vi "LL_GET Bucket.vi"(4 "Region":T1, 7 "GET Bucket Request Parameters":T9 {"max-keys" max=1000}, 8 "error in (no error)":errorcluster, 9 "Bucket":string, 11 "Headers":T8[](array[typedef])) -> (0 "error out":errorcluster, 1 "Call Result":T2, 3 "ListBucketResult":T3)   [LabVIEW 2015, in "LV Interface for Amazon S3.lvlib"]
doc: "This core implementation of the GET operation returns some or all (up to 1000) of the objects in a bucket. You can use the request parameters as selection criteria to return a subset of the objects in a bucket. You have direct access to HTTP headers, so you can use this VI to implement special requests or API calls not present in this toolkit."
uses:
  LV Interface for Amazon S3.lvlib
  Typedefs/AMZ_S3_API_GET Bucket Request Parameters.ctl
  Typedefs/AMZ_S3_HTTP Header-Value pair.ctl
  Typedefs/AMZ_S3_API_ListBucketResult.ctl
  Typedefs/AMZ_S3_API_ListBucketResult Content.ctl
  Typedefs/AMZ_S3_Storage Class.ctl
  Typedefs/AMZ_S3_API_Owner.ctl
  Typedefs/AMZ_S3_API_ListBucketResult CommonPrefix.ctl
  Typedefs/AMZ_S3_Call Results.ctl
  Typedefs/AMZ_S3_LocationConstraint.ctl
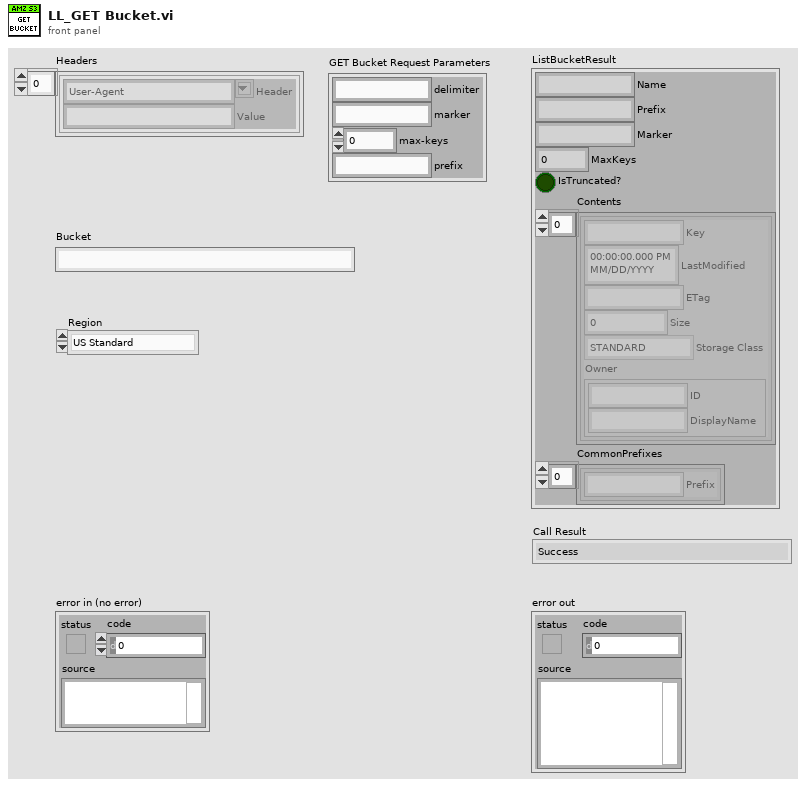
[diagram p1: front panel]
types:
  T1 = typedef "LV Interface for Amazon S3.lvlib/AMZ_S3_LocationConstraint.ctl" = enum16{"US Standard", "us-east-2", "us-west-1", "us-west-2", "ap-northeast-1", "ap-northeast-2", "ap-southeast-1", "ap-southeast-2", "ca-central-1", "eu-central-1", "eu-west-1", "eu-west-2", "sa-east-1"}
  T2 = typedef "LV Interface for Amazon S3.lvlib/AMZ_S3_Call Results.ctl" = enum16{"Success", "UndefinedError", "AccessDenied", "AccountProblem", "AmbiguousGrantByEmailAddress", "BadDigest", "BucketAlreadyExists", "BucketAlreadyOwnedByYou", "BucketNotEmpty", "CredentialsNotSupported", "CrossLocationLoggingProhibited", "EntityTooSmall", "EntityTooLarge", "ExpiredToken", "IllegalVersioningConfigurationException", "IncompleteBody", "IncorrectNumberOfFilesInPostRequest", "InlineDataTooLarge", "InternalError", "InvalidAccessKeyId", "InvalidAddressingHeader", "InvalidArgument", "InvalidBucketName", "InvalidDigest", "InvalidLocationConstraint", "InvalidPart", "InvalidPartOrder", "InvalidPayer", "InvalidPolicyDocument", "InvalidRange", "InvalidSecurity", "InvalidSOAPRequest", "InvalidStorageClass", "InvalidTargetBucketForLogging", "InvalidToken", "InvalidURI", "KeyTooLong", "MalformedACLError", "MalformedPOSTRequest", "MalformedXML", "MaxMessageLengthExceeded", "MaxPostPreDataLengthExceededError", "MetadataTooLarge", "MethodNotAllowed", "MissingAttachment", "MissingContentLength", "MissingRequestBodyError", "MissingSecurityElement", "MissingSecurityHeader", "NoLoggingStatusForKey", "NoSuchBucket", "NoSuchKey", "NoSuchUpload", "NoSuchVersion", "NotImplemented", "NotSignedUp", "OperationAborted", "PermanentRedirect", "PreconditionFailed", "Redirect", "RequestIsNotMultiPartContent", "RequestTimeout", "RequestTimeTooSkewed", "RequestTorrentOfBucketError", "SignatureDoesNotMatch", "SlowDown", "TemporaryRedirect", "TokenRefreshRequired", "TooManyBuckets", "UnexpectedContent", "UnresolvableGrantByEmailAddress", "UserKeyMustBeSpecified", "LabVIEWError"}
  T3 = typedef "LV Interface for Amazon S3.lvlib/AMZ_S3_API_ListBucketResult.ctl" = cluster{"Name":string, "Prefix":string, "Marker":string, "MaxKeys":u16, "IsTruncated?":bool, "Contents":T4[], "CommonPrefixes":T7[]}
  T4 = typedef "LV Interface for Amazon S3.lvlib/AMZ_S3_API_ListBucketResult Content.ctl" = cluster{"Key":string, "LastModified":timestamp, "ETag":string, "Size":u64, "Storage Class":T5, "Owner":T6}
  T5 = typedef "LV Interface for Amazon S3.lvlib/AMZ_S3_Storage Class.ctl" = enum16{"STANDARD", "REDUCED_REDUNDANCY"}
  T6 = typedef "LV Interface for Amazon S3.lvlib/AMZ_S3_API_Owner.ctl" = cluster{"ID":string, "DisplayName":string}
  T7 = typedef "LV Interface for Amazon S3.lvlib/AMZ_S3_API_ListBucketResult CommonPrefix.ctl" = cluster{"Prefix":string}
  T8 = typedef "LV Interface for Amazon S3.lvlib/AMZ_S3_HTTP Header-Value pair.ctl" = cluster{"Header":string, "Value":string}
  T9 = typedef "LV Interface for Amazon S3.lvlib/AMZ_S3_API_GET Bucket Request Parameters.ctl" = cluster{"delimiter":string, "marker":string, "max-keys":u16, "prefix":string}
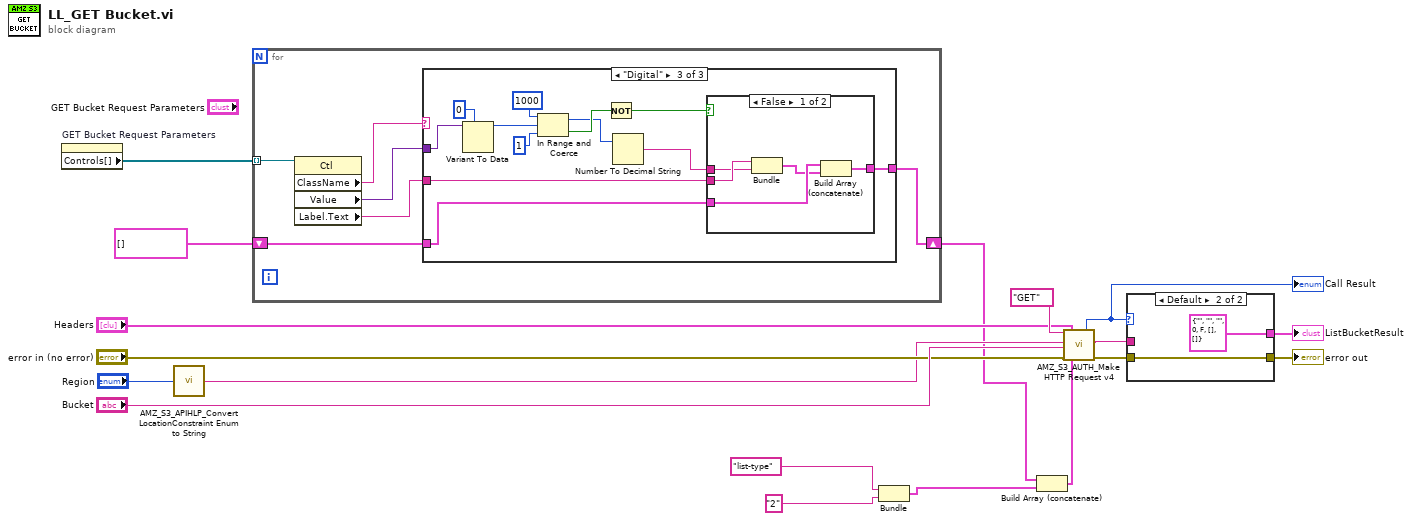
[diagram p0: block diagram]
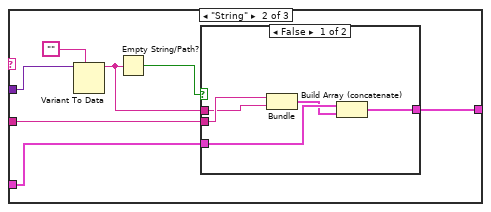
[diagram p3: hidden frame]
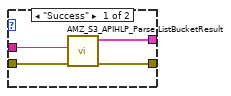
[diagram p6: hidden frame]
diagram:
  n1 = property on="GET Bucket Request Parameters" class="Clust (strict)"() -> ("Controls[]"=w10:refnum<vi>[])  [unwired: 2 in, 2 out]
  n2 = call "AMZ_S3_APIHLP_Convert LocationConstraint Enum to String.vi"("Location"="Region") -> ("Location String"=w6:string)  [unwired: 4 in]
  n3 = for {
    tunnel: w10 -> [w24] mode=indexing
    shift-right: [w19] -> w2
    shift-left: cluster{"item":string, "value":string}[] [] ("request parameters") -> [w21]
    n4 = property class="Ctl"(reference=w24) -> ("ClassName"=w23:string, "Value"=w22:variant, "Label.Text"=w20:string)  [unwired: 1 in, 2 out]
    n5 = case shown="\"Digital\"" w23 {
      tunnel: w22 -> [_ w31 w50]
      tunnel: w21 -> [w25 w29 w49]
      tunnel: w20 -> [_ w27 w48]
      tunnel: [w25 w26 w47] -> w19
      frame "False", Default {
      }
      frame "String" {
        n6 = Variant To Data(type="", Variant=w31) -> (data=w28:string)  [unwired: 1 in, 1 out]
        n7 = Empty String/Path?(string/path=w28) -> (empty?=w30:bool)
        n8 = case shown="False" w30 {
          tunnel: w29 -> [w35 w38]
          tunnel: w28 -> [w36 _]
          tunnel: w27 -> [w37 _]
          tunnel: [w33 w38] -> w26
          frame False {
            n9 = Bundle("Label.Text"=w37, w36) -> (w34:cluster{"Label.Text":string, string})  [unwired: 1 in]
            n10 = Build Array (concatenate)(w35, w34) -> (w33:cluster{"Label.Text":string, "value":string}[])
          }
          frame True {
          }
        }
      }
      frame "Digital" {
        n11 = Variant To Data(type=0, Variant=w50) -> (data=w41:i32)  [unwired: 1 in, 1 out]
        n12 = In Range and Coerce(upper limit=u16 1000, x=w41, lower limit=u16 1) -> (coerced(x)=w42:i32, In Range?=w43:bool)
        n13 = Not(x=w43) -> (.not. x?=w39:bool)
        n14 = Number To Decimal String(number=w42) -> (decimal integer string=w40:string)  [unwired: 1 in]
        n15 = case shown="False" w39 {
          tunnel: w49 -> [w53 w56]
          tunnel: w40 -> [w54 _]
          tunnel: w48 -> [w55 _]
          tunnel: [w51 w56] -> w47
          frame False {
            n16 = Bundle("Label.Text"=w55, w54) -> (w52:cluster{"Label.Text":string, string})  [unwired: 1 in]
            n17 = Build Array (concatenate)(w53, w52) -> (w51:cluster{"Label.Text":string, "value":string}[])
          }
          frame True {
          }
        }
      }
    }
  }
  n18 = Bundle("list-type", "2") -> (w3:cluster{string, string})  [unwired: 1 in]
  n19 = Build Array (concatenate)(w2, w3) -> (w1:cluster{"item":string, "value":string}[])
  n20 = call "AMZ_S3_AUTH_Make HTTP Request v4.vi"("HTTP-Verb"="GET", "Region"=w6, "Bucket"="Bucket", "error in"="error in (no error)", "request headers"="Headers", "request parameters"=w1) -> ("Call Result"=w16:T2, "response body"=w14:string, "error out"=w12:errorcluster)  [unwired: 10 in, 1 out]
  "Call Result" <- w16
  n21 = case shown="Default" w16 {
    tunnel: w14 -> [w60 _]
    tunnel: w12 -> [w59 w61]
    tunnel: [w58 T3 {"Name"="", "Prefix"="", "Marker"="", "MaxKeys"=0, "IsTruncated?"=FALSE, "Contents"=[], "CommonPrefixes"=[]} ("ListBucketResult")] -> w18
    tunnel: [w57 w61] -> w17
    frame "Success" {
      n22 = call "AMZ_S3_APIHLP_Parse ListBucketResult.vi"("error in (no error)"=w59, "Response body"=w60) -> ("error out"=w57:errorcluster, "ListBucketResult"=w58:T3)  [unwired: 8 in]
    }
    frame Default {
    }
  }
  "ListBucketResult" <- w18
  "error out" <- w17
